vi "FisherPaykel Serial Setup.vi"(7 "Debug":bool, 8 "error in (no error)":errorcluster, 11 "VISA Refnum in":refnum<visa-resource-name>) -> (0 "Error Out":errorcluster, 3 "VISA Refnum out":refnum<visa-resource-name>)   [LabVIEW 2016]
uses:
  <vilib>/Instr/_visa.llb/VISA Configure Serial Port (Instr).vi
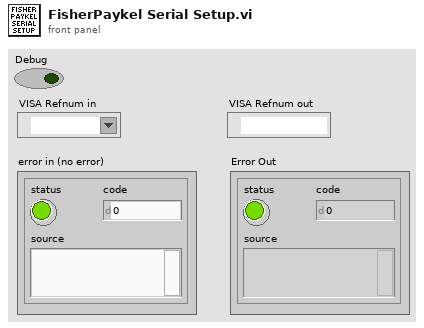
[diagram p1: front panel]
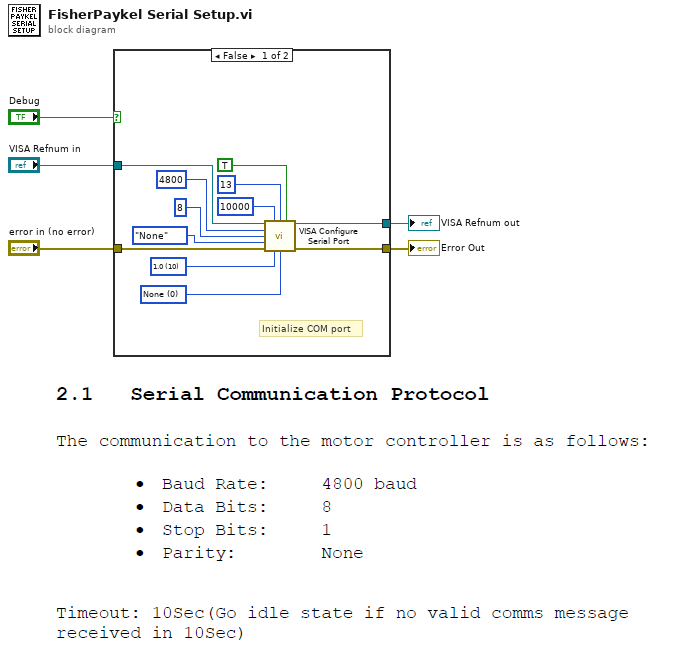
[diagram p0: block diagram]
diagram:
  n1 = case shown="False" "Debug" {
    tunnel: [w17 w19] -> w5
    tunnel: "error in (no error)" -> [w16 w18]
    tunnel: "VISA Refnum in" -> [w15 w19]
    tunnel: [w6 w18] -> w2
    frame False {
      w12 = u16 10 items=["1.0"=10, "1.5"=15, "2.0"=20] ("stop bits (10: 1 bit)")
      w11 = u16 0 items=["None", "XON/XOFF", "RTS/CTS", "XON/XOFF & RTS/CTS", "DTR/DSR", "XON/XOFF & DTR/DSR"] ("flow control (0:none)")
      # "Initialize COM port"
      n2 = call-poly "VISA Configure Serial Port"("VISA resource name"=w15, "timeout (10sec)"=u32 10000, "termination char\n(0xA = '\\n' = LF)"=u8 13 ("termination char\n(0xA = '\\n' = LF)"), "Enable Termination\nChar (T)"=TRUE ("Enable Termination\nChar (T)"), "baud rate (9600)"=u32 4800, "data bits (8)"=u16 8, "parity (0:none)"=enum16{"None", "Odd", "Even", "Mark", "Space"}."None", "error in (no error)"=w16, "stop bits (10: 1 bit)"=w12, "flow control (0:none)"=w11) -> ("VISA resource name out"=w17:refnum<visa-resource-name>, "error out"=w6:errorcluster)  [unwired: 4 in]
    }
    frame True {
    }
  }
  "VISA Refnum out" <- w5
  "Error Out" <- w2
